vi "SubVI_UI.vi"(8 "error in (no error)":errorcluster caption="err in", 11 "Q_data":T1) -> (0 "error out":errorcluster caption="err out")   [LabVIEW 2016]
uses:
  Ctrls/raw Q data.ctl
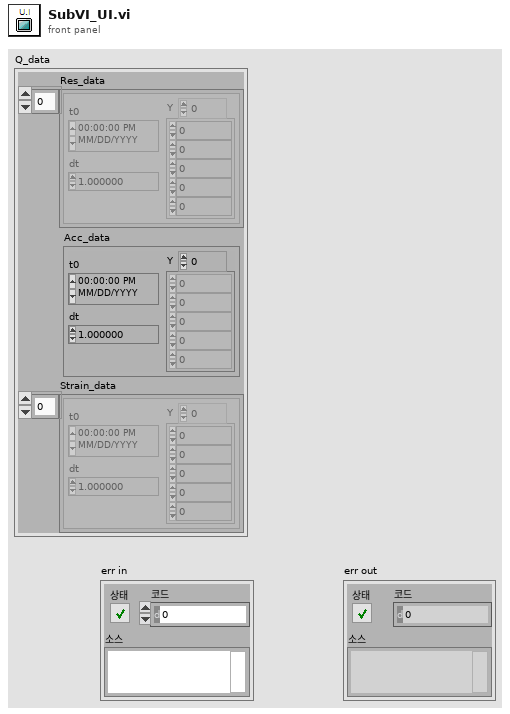
[diagram p1: front panel]
types:
  T1 = typedef "raw Q data.ctl" = cluster{"Res_data":waveform(dbl)[], "Acc_data":waveform(dbl), "Strain_data":waveform(dbl)[]}
  T2 = typedef "ui ctrl ref2.ctl" = cluster{"Trigger cm":refnum<vi>, "Speed In/s":refnum<vi>, "Start / Stop":refnum<vi>, "Test Information":refnum<vi>, "STATUS":refnum<vi>, "Result Table":refnum<vi>, "Acc. & Strian Result":refnum<vi>, "Curr Resistor (Ω)":refnum<vi>, "Scroll":refnum<vi>, "All Data Graph":refnum<vi>, "Acc. Graph":refnum<vi>}
  T3 = typedef "Total data.ctl" = cluster{"Raw Data":T1, "Resister result data":T4, "Result Table update":cluster{"Num":u32[], "Resister 1~5":u8[][], "Resister 6~10":u8[][], "Resister 11~15":u8[][]}, "Strain Data":cluster{"Strain 1":dbl, "Strain 2":dbl, "Strain 3":dbl, "Strain 4":dbl}, "Acc Result":cluster{"Acc Peak":dbl, "Acc time":dbl, "Acc area":dbl}, "STATUS":cluster{"status":string, "all_fail":bool, "emg":bool, "cycle":u16, "file name":string}, "Speed":dbl, "Acc peak time":dbl, "Max Strain":dbl, "Resistor at peak":cluster{"[0]":dbl, "[1]":dbl, "[2]":dbl, "[3]":dbl, "[4]":dbl, "[5]":dbl, "[6]":dbl, "[7]":dbl, "[8]":dbl, "[9]":dbl, "[10]":dbl, "[11]":dbl, "[12]":dbl, "[13]":dbl, "[14]":dbl}, "Acc peak index":u32, "time":string, "Cycle finish":bool, "Resistor at ini":cluster{"[0]":dbl, "[1]":dbl, "[2]":dbl, "[3]":dbl, "[4]":dbl, "[5]":dbl, "[6]":dbl, "[7]":dbl, "[8]":dbl, "[9]":dbl, "[10]":dbl, "[11]":dbl, "[12]":dbl, "[13]":dbl, "[14]":dbl}}
  T4 = typedef "raw data type.ctl" = cluster{"Resistor values":cluster{"[0]":dbl, "[1]":dbl, "[2]":dbl, "[3]":dbl, "[4]":dbl, "[5]":dbl, "[6]":dbl, "[7]":dbl, "[8]":dbl, "[9]":dbl, "[10]":dbl, "[11]":dbl, "[12]":dbl, "[13]":dbl, "[14]":dbl}, "Resistor tables":u8[], "Pass Fails":bool[]}
  T5 = cluster{"status":string, "all_fail":bool, "emg":bool, "cycle":u16, "file name":string, "Total Cycle":u32}
  T6 = cluster{"[0]":dbl, "[1]":dbl, "[2]":dbl, "[3]":dbl, "[4]":dbl, "[5]":dbl, "[6]":dbl, "[7]":dbl, "[8]":dbl, "[9]":dbl, "[10]":dbl, "[11]":dbl, "[12]":dbl, "[13]":dbl, "[14]":dbl}
  T7 = cluster{"Num":u32[], "Resister 1~5":u8[][], "Resister 6~10":u8[][], "Resister 11~15":u8[][]}
  T8 = cluster{"status":string, "all_fail":bool, "emg":bool, "cycle":u16, "file name":string}
  T9 = cluster{"Test Information":cluster{"date":string, "custom":string, "oper":string, "package":string, "pkg side":string, "solder":string, "brd side":string, "paste":string, "reflow":string}, "Sensor Set":cluster{"Accelerometer":cluster{"Sensitivity(mV/g)":dbl}, "Strain Guage":cluster{"Ch.":dbl[], "Gage factor":dbl[], "Resistance":dbl[], "Poisson ratio":dbl[]}}, "Resistor Set":cluster{"Criterion Level":dbl, "Res. Set":cluster{"Res. Ch":dbl, "Res. Active":bool, "Res Initial":dbl}[]}, "Test Stop Condition":cluster{"Test cycle":u16, "Fail number in a cycle":u16, "Fail factor":cluster{"Duration":u16, "Fail No.":u16}}, "Acceleration Condition ":cluster{"Shock duration pecent [%]":u16, "Filter cutoff freq":u32}, "Save":cluster{"Save Path":path, "File Name":string}}
  T10 = cluster{"Acc Peak":dbl, "Acc time":dbl, "Acc area":dbl}
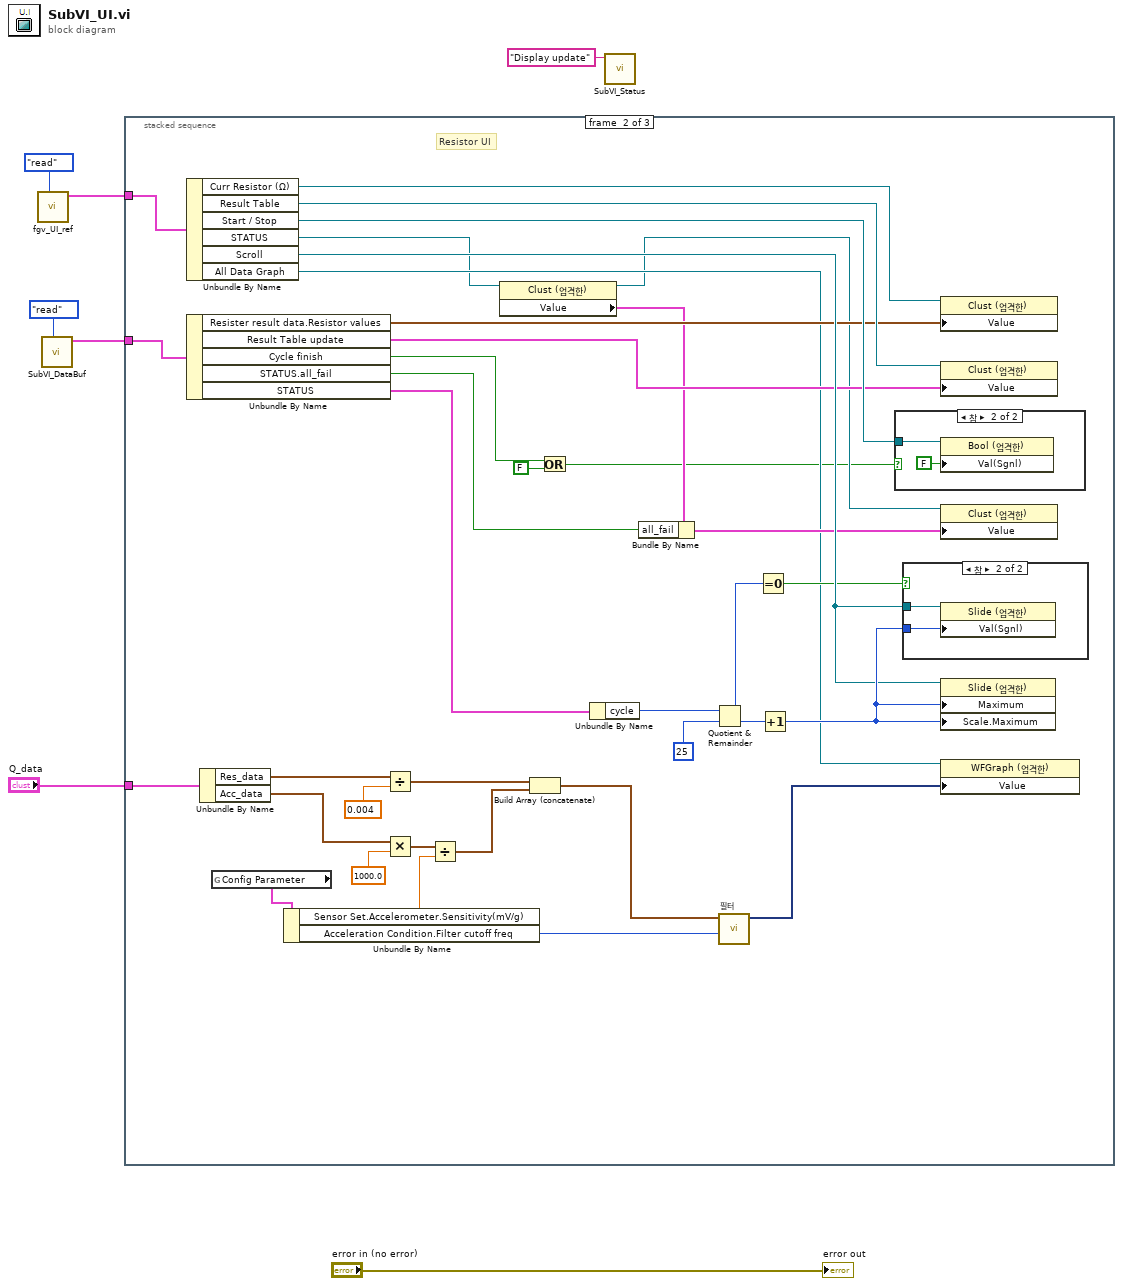
[diagram p0: block diagram]
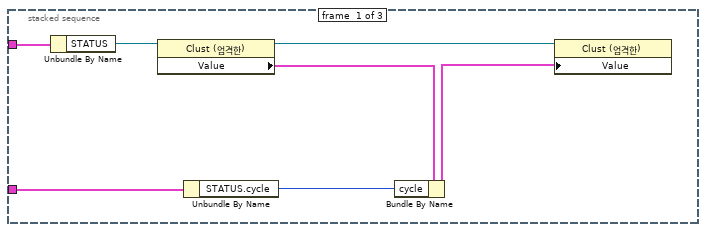
[diagram p2: hidden frame]
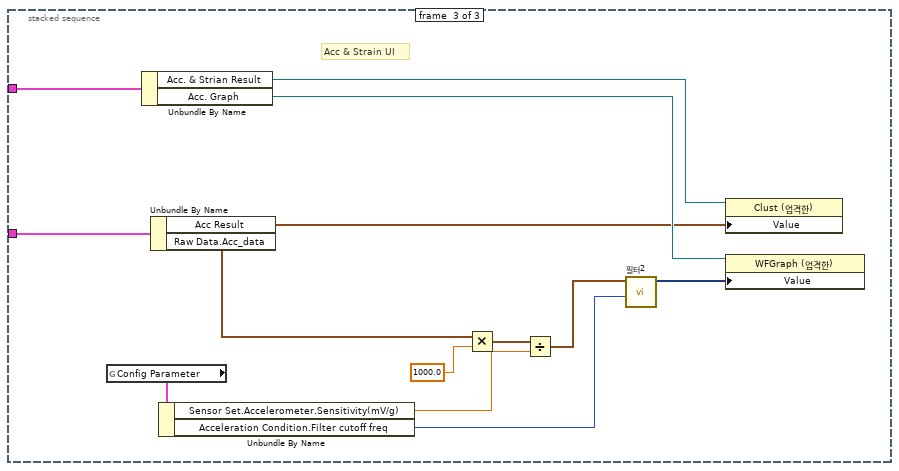
[diagram p5: hidden frame]
diagram:
  n1 = call "fgv_UI_ref.vi"("cmd"=enum16{"write", "read"}."read") -> ("ui ref out"=w5:T2)  [unwired: 10 in]
  n2 = call "SubVI_DataBuf.vi"("cmd"=enum16{"ini", "write", "read"}."read") -> ("Total data 2"=w3:T3)  [unwired: 9 in, 1 out]
  n3 = stacked-sequence {
    tunnel: w5 -> [w14 w41 w66]
    tunnel: w3 -> [w13 w40 w65]
    tunnel: "Q_data" -> [_ w36 _]
    frame #0 {
      n4 = Unbundle By Name(w14) -> ("STATUS"=w12:refnum<vi>)
      n5 = property class="Clust (엄격한)"(reference=w12) -> (reference out=w9:refnum<vi>, "Value"=w11:T5)  [unwired: 1 in, 1 out]
      n6 = Unbundle By Name(w13) -> ("STATUS.cycle"=w8:u16)
      n7 = Bundle By Name(cluster=w11, "cycle"=w8) -> (w10:T5)
      n8 = property class="Clust (엄격한)"(reference=w9, "Value"=w10) -> ()  [unwired: 1 in, 2 out]
    }
    frame #1 {
      # "Resistor UI"
      n9 = Unbundle By Name(w41) -> ("Curr Resistor (Ω)"=w42:refnum<vi>, "Result Table"=w43:refnum<vi>, "Start / Stop"=w51:refnum<vi>, "STATUS"=w24:refnum<vi>, "Scroll"=w49:refnum<vi>, "All Data Graph"=w37:refnum<vi>)
      n10 = Unbundle By Name(w40) -> ("Resister result data.Resistor values"=w39:T6, "Result Table update"=w38:T7, "Cycle finish"=w20:bool, "STATUS.all_fail"=w21:bool, "STATUS"=w22:T8)
      n11 = Unbundle By Name(w36) -> ("Res_data"=w34:waveform(dbl)[], "Acc_data"=w28:waveform(dbl))
      n12 = global read "글로벌_Config Parameter.vi" "Config Parameter"() -> (w32:T9)
      n13 = Unbundle By Name(w32) -> ("Sensor Set.Accelerometer.Sensitivity(mV/g)"=w29:dbl, "Acceleration Condition.Filter cutoff freq"=w15:u32)
      n14 = Divide(x=w34, y=0.004) -> (x/y=w33:waveform(dbl)[])
      n15 = Multiply(x=w28, y=1000.0) -> (x*y=w30:waveform(dbl))
      n16 = Divide(x=w30, y=w29) -> (x/y=w27:waveform(dbl))
      n17 = property class="Clust (엄격한)"(reference=w24) -> (reference out=w23:refnum<vi>, "Value"=w25:T5)  [unwired: 1 in, 1 out]
      n18 = Build Array (concatenate)(w33, w27) -> (w17:waveform(dbl)[])
      n19 = Or(x=w20, y=FALSE) -> (x .or. y?=w19:bool)
      n20 = Unbundle By Name(w22) -> ("cycle"=w26:u16)
      n21 = Bundle By Name(cluster=w25, "all_fail"=w21) -> (w44:T5)
      n22 = Quotient & Remainder(x=w26, y=i16 25) -> (x-y*floor(x/y)=w45:u16, floor(x/y)=w46:u16)
      n23 = call "필터"("Lower Cut-Off"=w15, "Signal"=w17) -> ("Filtered Signal"=w16:dynamicdata)  [unwired: 8 in, 1 out]
      n24 = Equal To 0?(x=w45) -> (x = 0?=w48:bool)
      n25 = Increment(x=w46) -> (x+1=w50:u16)
      n26 = case shown="참" w19 {
        tunnel: w51 -> [_ w53]
        frame False {
        }
        frame True {
          n27 = property class="Bool (엄격한)"(reference=w53, "Val(Sgnl)"=FALSE ("값(신호)")) -> ()  [unwired: 1 in, 2 out]
        }
      }
      n28 = case shown="참" w48 {
        tunnel: w49 -> [_ w55]
        tunnel: w50 -> [_ w54]
        frame False {
        }
        frame True {
          n29 = property class="Slide (엄격한)"(reference=w55, "Val(Sgnl)"=w54) -> ()  [unwired: 1 in, 2 out]
        }
      }
      n30 = property class="Clust (엄격한)"(reference=w42, "Value"=w39) -> ()  [unwired: 1 in, 2 out]
      n31 = property class="Clust (엄격한)"(reference=w43, "Value"=w38) -> ()  [unwired: 1 in, 2 out]
      n32 = property class="Clust (엄격한)"(reference=w23, "Value"=w44) -> ()  [unwired: 1 in, 2 out]
      n33 = property on="프로퍼티 노드" class="Slide (엄격한)"(reference=w49, "Maximum"=w50, "Scale.Maximum"=w50) -> ()  [unwired: 1 in, 2 out]
      n34 = property class="WFGraph (엄격한)"(reference=w37, "Value"=w16) -> ()  [unwired: 1 in, 2 out]
    }
    frame #2 {
      # "Acc & Strain UI"
      n35 = global read "글로벌_Config Parameter.vi" "Config Parameter"() -> (w63:T9)
      n36 = Unbundle By Name(w66) -> ("Acc. & Strian Result"=w67:refnum<vi>, "Acc. Graph"=w68:refnum<vi>)
      n37 = Unbundle By Name(w65) -> ("Acc Result"=w64:T10, "Raw Data.Acc_data"=w59:waveform(dbl))
      n38 = Unbundle By Name(w63) -> ("Sensor Set.Accelerometer.Sensitivity(mV/g)"=w60:dbl, "Acceleration Condition.Filter cutoff freq"=w56:u32)
      n39 = Multiply(x=w59, y=1000.0) -> (x*y=w61:waveform(dbl))
      n40 = Divide(x=w61, y=w60) -> (x/y=w58:waveform(dbl))
      n41 = call "필터2"("Lower Cut-Off"=w56, "Signal"=w58) -> ("Filtered Signal"=w57:dynamicdata)  [unwired: 8 in, 1 out]
      n42 = property class="Clust (엄격한)"(reference=w67, "Value"=w64) -> ()  [unwired: 1 in, 2 out]
      n43 = property class="WFGraph (엄격한)"(reference=w68, "Value"=w57) -> ()  [unwired: 1 in, 2 out]
    }
  }
  n44 = call "SubVI_Status.vi"("info_str"="Display update") -> ()  [unwired: 10 in, 1 out]
  "error out" <- "error in (no error)"
